vi "Win_LSE_loop.vi"(0 "N":dbl, 1 "dx/dt":dbl, 2 "x(t)":dbl, 3 "u(t)":dbl, 4 "error in (no error)":errorcluster) -> (5 "\\theta(t)":T1, 6 "error out":errorcluster)   [LabVIEW 2021]
uses:
  <vilib>/Analysis/Matrix/Datatypes/RealMatrix.ctl
  <vilib>/Analysis/3filter.llb/Filter Passband Type.ctl
  <vilib>/Analysis/Matrix/NI_Matrix.lvlib
  <vilib>/ptbypt/NI_PtbyPt.lvlib
  <vilib>/Analysis/NI_AALBase.lvlib
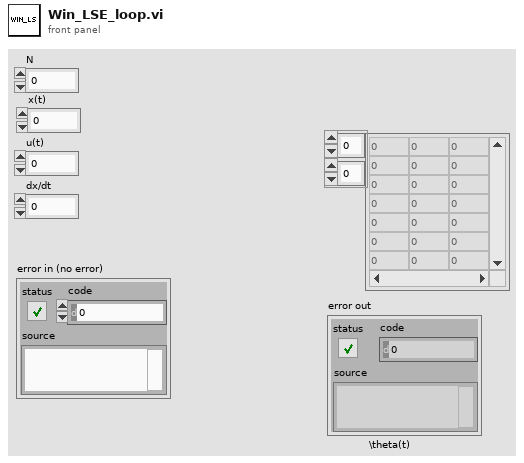
[diagram p1: front panel]
types:
  T1 = typedef "NI_Matrix.lvlib/RealMatrix.ctl" = dbl[][]
  T2 = typedef "NI_AALBase.lvlib/Filter Passband Type.ctl" = enum32{"Lowpass", "Highpass", "Bandpass", "Bandstop"}
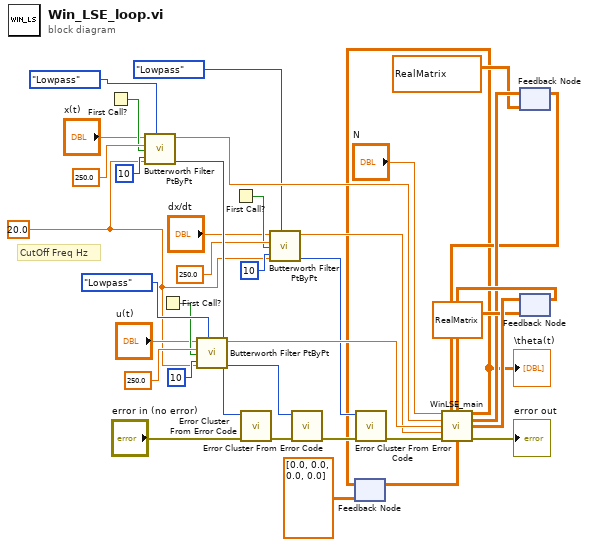
[diagram p0: block diagram]
diagram:
  w3 = 20.0 ("high cutoff freq: fh")
  # "CutOff Freq Hz"
  n1 = First Call?() -> (First Call?: T/F=w26:bool)
  n2 = call <vilib>:"Butterworth Filter PtByPt.vi"("initialize"=w26, "order"=10, "filter type"=Filter_Passband_Type."Lowpass", "low cutoff freq: fl"=w3, "sampling freq: fs"=250.0, "x"="x(t)") -> ("error"=w24:i32, "Filtered x"=w21:dbl)  [unwired: 3 in]
  n3 = First Call?() -> (First Call?: T/F=w18:bool)
  n4 = call <vilib>:"Butterworth Filter PtByPt.vi"("initialize"=w18, "order"=10, "filter type"=Filter_Passband_Type."Lowpass", "low cutoff freq: fl"=w3, "sampling freq: fs"=250.0, "x"="u(t)") -> ("error"=w16:i32, "Filtered x"=w14:dbl)  [unwired: 3 in]
  n5 = First Call?() -> (First Call?: T/F=w10:bool)
  n6 = call <vilib>:"Error Cluster From Error Code.vi"("error in (no error)"="error in (no error)", "error code (0)"=w24) -> ("error out"=w13:errorcluster)  [unwired: 7 in]
  n7 = call <vilib>:"Butterworth Filter PtByPt.vi"("initialize"=w10, "order"=10, "filter type"=Filter_Passband_Type."Lowpass", "low cutoff freq: fl"=w3, "sampling freq: fs"=250.0, "x"="dx/dt") -> ("error"=w8:i32, "Filtered x"=w6:dbl)  [unwired: 3 in]
  n8 = call <vilib>:"Error Cluster From Error Code.vi"("error in (no error)"=w13, "error code (0)"=w16) -> ("error out"=w5:errorcluster)  [unwired: 7 in]
  n9 = feedback #1(T1 [[0.0], [0.0], [0.0], [0.0]] ("\\theta(t)")) -> (w30:T1)
  n10 = call <vilib>:"Error Cluster From Error Code.vi"("error in (no error)"=w5, "error code (0)"=w8) -> ("error out"=w4:errorcluster)  [unwired: 7 in]
  n11 = feedback #2(T1 [[0.0, 0.0, 0.0, 0.0, 0.0, 0.0, 0.0, 0.0, 0.0, 0.0, 0.0, 0.0, 0.0, 0.0, 0.0, 0.0, 0.0, 0.0, 0.0, 0.0, 0.0, 0.0, 0.0, 0.0, 0.0, 0.0, 0.0, 0.0, 0.0, 0.0, 0.0, 0.0, 0.0, 0.0, 0.0, 0.0, 0.0, 0.0, 0.0, 0.0, 0.0, 0.0, 0.0, 0.0, 0.0, 0.0, 0.0, 0.0, 0.0, 0.0, 0.0, 0.0, 0.0, 0.0, 0.0, 0.0, 0.0, 0.0, 0.0, 0.0, 0.0, 0.0, 0.0, 0.0, 0.0, 0.0, 0.0, 0.0, 0.0, 0.0, 0.0, 0.0, 0.0, 0.0, 0.0, 0.0, 0.0, 0.0, 0.0, 0.0, 0.0, 0.0, 0.0, 0.0, 0.0, 0.0, 0.0, 0.0, 0.0, 0.0, 0.0, 0.0, 0.0, 0.0, 0.0, 0.0, 0.0, 0.0, 0.0, 0.0]] ("Omega(t)")) -> (w32:T1)
  n12 = feedback #3(T1 [[0.0, 0.0, 0.0, 0.0, 0.0, 0.0, 0.0, 0.0, 0.0, 0.0, 0.0, 0.0, 0.0, 0.0, 0.0, 0.0, 0.0, 0.0, 0.0, 0.0, 0.0, 0.0, 0.0, 0.0, 0.0, 0.0, 0.0, 0.0, 0.0, 0.0, 0.0, 0.0, 0.0, 0.0, 0.0, 0.0, 0.0, 0.0, 0.0, 0.0, 0.0, 0.0, 0.0, 0.0, 0.0, 0.0, 0.0, 0.0, 0.0, 0.0, 0.0, 0.0, 0.0, 0.0, 0.0, 0.0, 0.0, 0.0, 0.0, 0.0, 0.0, 0.0, 0.0, 0.0, 0.0, 0.0, 0.0, 0.0, 0.0, 0.0, 0.0, 0.0, 0.0, 0.0, 0.0, 0.0, 0.0, 0.0, 0.0, 0.0, 0.0, 0.0, 0.0, 0.0, 0.0, 0.0, 0.0, 0.0, 0.0, 0.0, 0.0, 0.0, 0.0, 0.0, 0.0, 0.0, 0.0, 0.0, 0.0, 0.0]] ("y(t)")) -> (w35:T1)
  n13 = call "WinLSE_main.vi"("N"="N", "Omega(t-1)"=w32, "y(t-1)"=w35, "x(t)"=w21, "u(t)"=w14, "dx/dt"=w6, "error in (no error)"=w4, "\\theta(t-1)"=w30) -> ("\\theta(t)"=w2:T1, "Omega(t)"=w33:T1, "y(t)"=w36:T1, "error out"=→"error out":errorcluster)  [unwired: 4 in]
  "\\theta(t)" <- w2
  n14 = feedback-in #1(w2) -> ()
  n15 = feedback-in #2(w33) -> ()
  n16 = feedback-in #3(w36) -> ()
